vi "Auto Align With Limelight.vi"(0 "Robot Velocities In":T3) -> (7 "Robot Velocities Out":T3, 8 "Rotational Velocity":dbl format="%.2f")   [LabVIEW 2020]
uses:
  Type Definitions/Data/Robot Velocities.ctl
  <vilib>/Rock Robotics/WPI/ThirdParty/Phoenix-LabVIEW/Pigeon IMU/CTRE_PigeonIMU_DeviceRef.ctl
  <vilib>/Rock Robotics/WPI/ThirdParty/Phoenix-LabVIEW/Pigeon IMU/CTRE_PigeonIMU_ConnectionType.ctl
  <vilib>/Rock Robotics/Network Tables/NT Read Number.vi
  <vilib>/Rock Robotics/WPI/ThirdParty/Phoenix-LabVIEW/Pigeon IMU/CTRE_PigeonIMU_GetYPR.vi
panel:
  in  "PigeonIMUDevRef":T1={"DeviceStatus"={"status"=FALSE, "code"=0, "source"=""}, "Device Number"=0, "Type"=352321536, "Device ID"=0, "Handle"=0, "UsageFrame"=0, "Library Path"=path ""} {"Type" items=["CAN"=352321536, "TalonSRX"=33554432]}
  in  "FeedFwd Value":dbl format="%.2f"
  out "Err/Out Chart":cluster{dbl, dbl}(graph)
  out "SP/PV Chart":cluster{"setpoint":dbl, "process variable":dbl}(graph)
  in  "PID gains":T4={"proportional gain (Kp)"=1.0, "integral time (Ki)"=0.0, "derivative time (Kd)"=0.0} {"derivative time (Kd)" format="%.3f"; "integral time (Ki)" format="%.3f"; "proportional gain (Kp)" format="%.3f"}
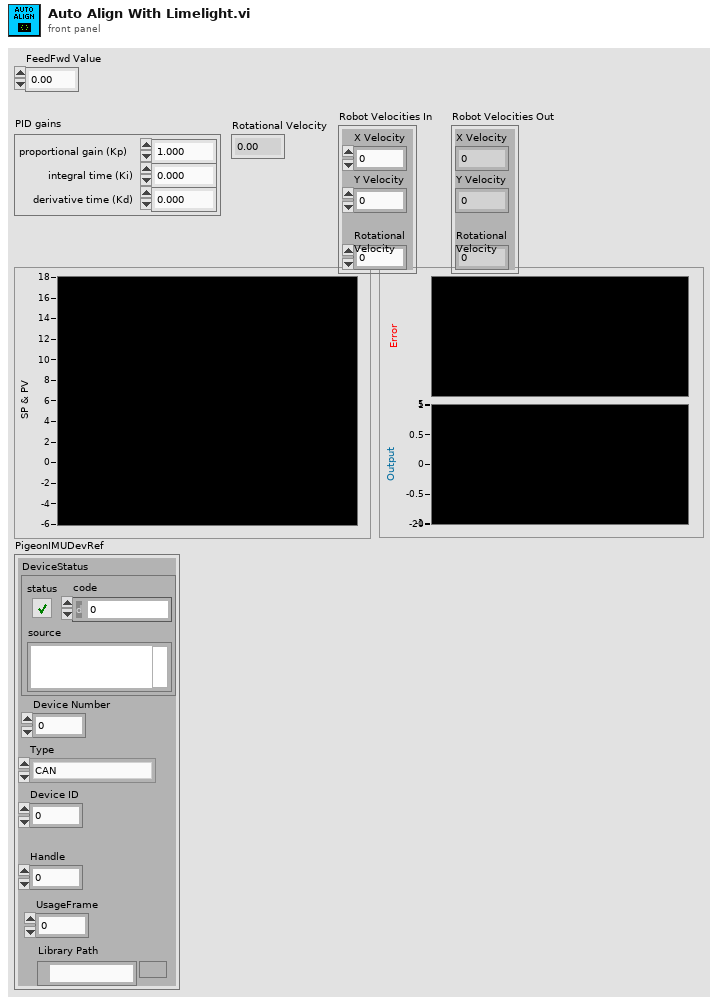
[diagram p1: front panel]
types:
  T1 = typedef "CTRE_PigeonIMU_DeviceRef.ctl" = cluster{"DeviceStatus":errorcluster, "Device Number":u8, "Type":T2, "Device ID":u32, "Handle":u64, "UsageFrame":u32, "Library Path":path}
  T2 = typedef "CTRE_PigeonIMU_ConnectionType.ctl" = u32
  T3 = typedef "Robot Velocities.ctl" = cluster{"X Velocity":dbl, "Y Velocity":dbl, "Rotational \nVelocity":dbl}
  T4 = cluster{"proportional gain (Kp)":dbl, "integral time (Ki)":dbl, "derivative time (Kd)":dbl}
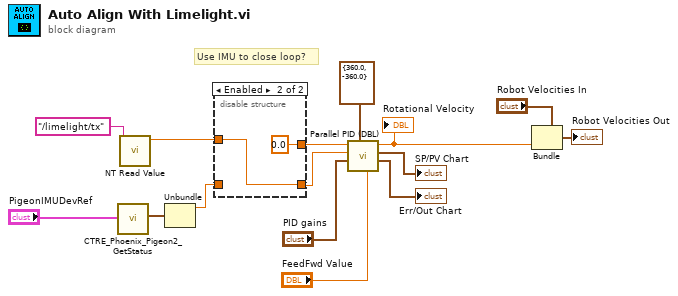
[diagram p0: block diagram]
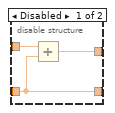
[diagram p2: hidden frame]
diagram:
  # "Use IMU to close loop?"
  n1 = call-poly <vilib>:"CTRE_Phoenix_Pigeon2_GetStatus.vi"("PigeonIMUDevRef"="PigeonIMUDevRef") -> ("Yaw Pitch Roll"=w5:cluster{"Yaw":dbl, "Pitch":dbl, "Roll":dbl})  [unwired: 8 in, 2 out]
  n2 = call-poly <vilib>:"NT Read Value.vi"("name"="/limelight/tx" ("Name")) -> ("value"=w4:dbl)  [unwired: 8 in, 2 out]
  n3 = Unbundle(w5) -> ("Yaw"=w2:dbl)  [unwired: 2 out]
  n4 = disable-structure shown="Enabled" {
    disable-tunnel: w4 -> [w18 w19]
    disable-tunnel: [w17 0.0 ("setpoint")] -> w3
    disable-tunnel: w2 -> [w16 _]
    disable-tunnel: [w16 w19] -> w1
    frame Disabled {
      n5 = Add(x=w18, y=w16) -> (x+y=w17:dbl)
    }
    frame Enabled {
    }
  }
  n6 = call <vilib>:"Parallel PID (DBL).vi"("FeedFwd Value"="FeedFwd Value", "output range"=cluster{"high":dbl, "low":dbl} {"high"=360.0, "low"=-360.0}, "PID gains"="PID gains", "process variable"=w1, "setpoint"=w3) -> ("Err/Out Chart"=→"Err/Out Chart":cluster{dbl, dbl}, "SP/PV Chart"=→"SP/PV Chart":cluster{"setpoint":dbl, "process variable":dbl}, "output"=w9:dbl)  [unwired: 3 in, 1 out]
  "Rotational Velocity" <- w9
  n7 = Bundle(cluster="Robot Velocities In", "Rotational \nVelocity"=w9) -> (→"Robot Velocities Out":T3)  [unwired: 2 in]
